vi "GeneralSettingsConfigure.vi"(11 "Email Notification Cluster in":T1) -> (3 "Email Notification Cluster out":T1)   [LabVIEW 2011]
uses:
  Controls/Ping address and email notify.ctl
panel:
  in  "Email Notification Settings":T1
  in  "Cancel Button":bool
  in  "OK Button":bool
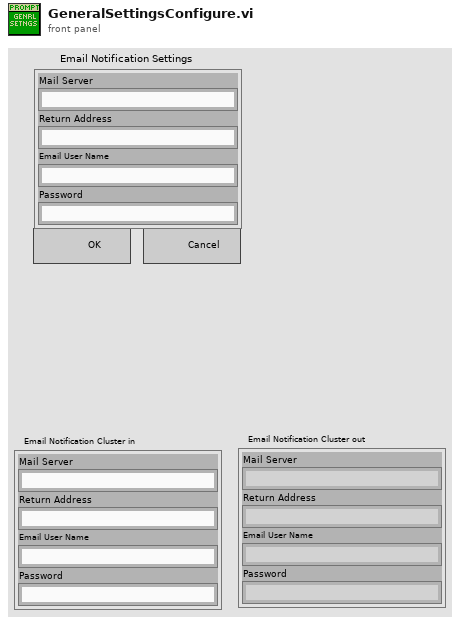
[diagram p1: front panel]
types:
  T1 = typedef "Ping address and email notify.ctl" = cluster{"Mail Server":string, "Return Address":string, "Email User Name":string, "Password":string}
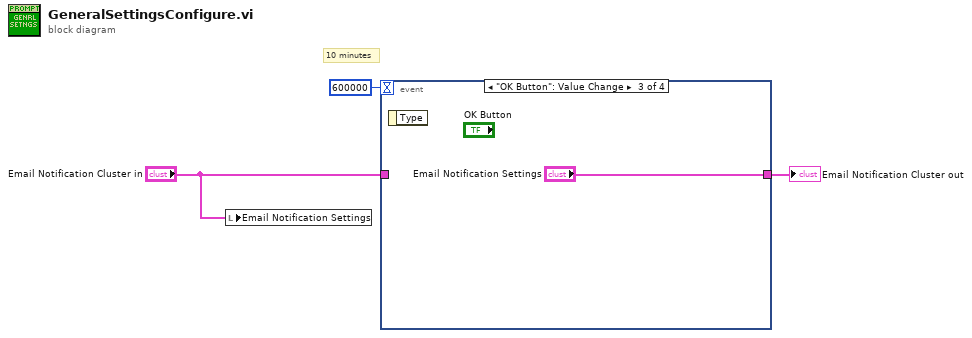
[diagram p0: block diagram]
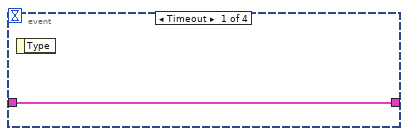
[diagram p2: hidden frame]
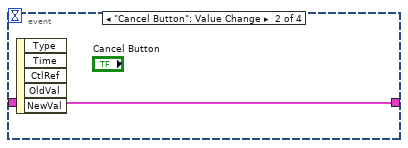
[diagram p3: hidden frame]
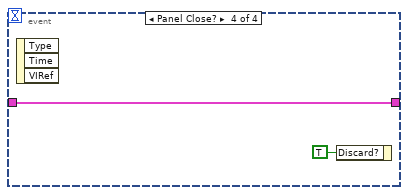
[diagram p4: hidden frame]
diagram:
  # "10 minutes"
  n1 = local write "Email Notification Settings"("Email Notification Cluster in") -> ()
  n2 = event shown="[2] \"OK Button\": Value Change" {
    selector: _ -> [_ _ _ _]
    dyn-events: _ -> [_ _ _ _]
    timeout: 600000 -> [_ _ _ _]
    tunnel: "Email Notification Cluster in" -> [w4 w5 _ w7]
    tunnel: [w4 w5 "Email Notification Settings" w7] -> w2
    event Timeout {
      n3 = event-data() -> ()  [unwired: 1 in, 1 out]
    }
    event "Cancel Button": Value Change {
      n4 = event-data() -> ()  [unwired: 1 in, 5 out]
    }
    event "OK Button": Value Change {
      n5 = event-data() -> ()  [unwired: 1 in, 1 out]
    }
    event Panel Close? {
      n6 = event-data() -> ()  [unwired: 1 in, 3 out]
      n7 = event-data("Discard?"=TRUE) -> ()  [unwired: 1 in, 1 out]
    }
  }
  "Email Notification Cluster out" <- w2
